vi "CRYGet Digital Port Array.vi"(11 "Dig I/O Ports":T1(array[cluster])) -> (3 "Digital Port Array":cluster{"String":string, "Value":ext}[](array[cluster]))   [LabVIEW 2013]
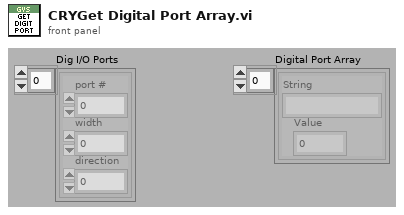
[diagram p1: front panel]
types:
  T1 = cluster{"port #":i16, "width":i16, "direction":i32}[]
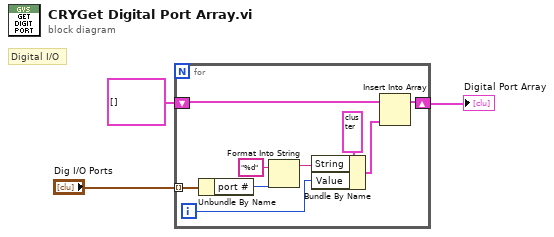
[diagram p0: block diagram]
diagram:
  # "Digital I/O"
  n1 = for {
    shift-right: [w12] -> w2
    shift-left: cluster{"String":string, "Value":ext}[] [] -> [w11]
    tunnel: "Dig I/O Ports" -> [w6] mode=indexing
    i -> [w4]
    n2 = Unbundle By Name(w6) -> ("port #"=w5:i16)
    n3 = Format Into String(format string="%d", w5) -> (resulting string=w9:string)  [unwired: 2 in, 1 out]
    n4 = Bundle By Name(cluster=cluster{"String":string, "Value":ext} {"String"="", "Value"=0.0}, "String"=w9, "Value"=w4) -> (w7:cluster{"String":string, "Value":ext})
    n5 = Insert Into Array(array=w11, new element=w7) -> (w12:cluster{"String":string, "Value":ext}[])  [unwired: 1 in]
  }
  "Digital Port Array" <- w2
